vi "Setup JJ IV.vi"(4 "Channel Name (1)":u16(ring)=1 items=["1"=1, "2"=2, "3"=3, "4"=4], 5 "VISA resource name":refnum<visa-resource-name>="GPIB0::1::INSTR", 7 "End time S":dbl=0.000105, 8 "error in (no error)":errorcluster, 9 "Ramp time S":dbl=0.01, 10 "Delay time S":dbl=0.01, 11 "Sampling Frequency (Hz)":u64=10000000 format="%^.2e") -> (0 "error out":errorcluster)   [LabVIEW 2021]
uses:
  <instrlib>/Tektronix AWG 5000 7000 Series/Public/Configure/Channel/Assign Output Waveform (From Waveform List).vi
  <instrlib>/Tektronix AWG 5000 7000 Series/Public/Configure/Configure Output Timing (Sampling Frequency).vi
  <instrlib>/Tektronix AWG 5000 7000 Series/Tektronix AWG 5000 7000 Series.lvlib
panel:
  in  "Jump height over Vpp":dbl=0.05
  in  "Ramp time S 2":dbl=0.0005
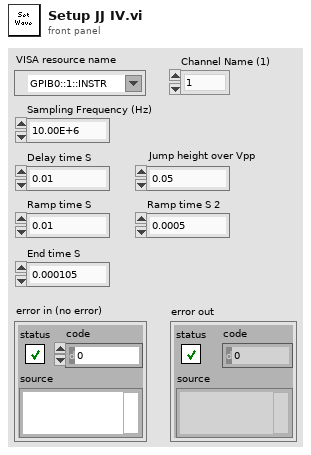
[diagram p1: front panel]
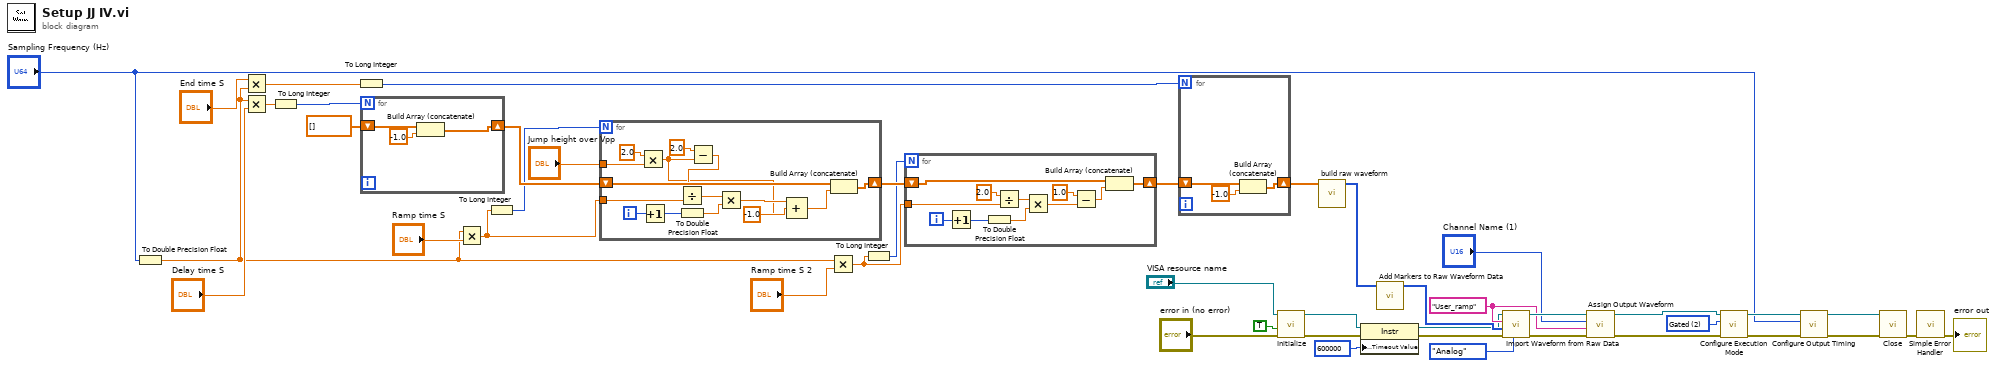
[diagram p0: block diagram]
diagram:
  w21 = u16 2 items=["Continuous", "Triggered", "Gated", "Sequence", "Triggered Continuous"] ("Execution Mode (0 : Continuous)")
  w23 = "User_ramp" ("Waveform Name")
  n1 = To Double Precision Float(number="Sampling Frequency (Hz)") -> (double precision float=w9:dbl)
  n2 = Multiply(x="End time S", y=w9) -> (x*y=w26:dbl)
  n3 = Multiply(x=w9, y="Delay time S") -> (x*y=w27:dbl)
  n4 = To Long Integer(number=w27) -> (32bit integer=w19:i32)
  n5 = To Long Integer(number=w26) -> (32bit integer=w2:i32)
  n6 = for {
    N: w19 -> [_]
    shift-right: [w46] -> w32
    shift-left: dbl[] [] -> [w47]
    n7 = Build Array (concatenate)(w47, -1.0) -> (w46:dbl[])
  }
  n8 = Multiply(x=w9, y="Ramp time S") -> (x*y=w5:dbl)
  n9 = To Long Integer(number=w5) -> (32bit integer=w18:i32)
  n10 = for {
    N: w18 -> [_]
    shift-right: [w55] -> w7
    shift-left: w32 -> [w57]
    tunnel: w5 -> [w54]
    tunnel: "Jump height over Vpp" -> [w51]
    i -> [w61]
    n11 = Multiply(x=2.0, y=w51) -> (x*y=w48:dbl)
    n12 = Increment(x=w61) -> (x+1=w60:i32)
    n13 = To Double Precision Float(number=w60) -> (double precision float=w53:dbl)
    n14 = Subtract(x=2.0, y=w48) -> (x-y=w49:dbl)
    n15 = Divide(x=w49, y=w54) -> (x/y=w62:dbl)
    n16 = Multiply(x=w62, y=w53) -> (x*y=w59:dbl)
    n17 = Compound Arithmetic op=ADD(w59, -1.0 ("y"), w48) -> (w56:dbl)
    n18 = Build Array (concatenate)(w57, w56) -> (w55:dbl[])
  }
  n19 = Multiply(x=w9, y="Ramp time S 2") -> (x*y=w4:dbl)
  n20 = To Long Integer(number=w4) -> (32bit integer=w3:i32)
  n21 = for {
    N: w3 -> [_]
    shift-right: [w72] -> w6
    shift-left: w7 -> [w73]
    tunnel: w4 -> [w71]
    i -> [w69]
    n22 = Increment(x=w69) -> (x+1=w68:i32)
    n23 = To Double Precision Float(number=w68) -> (double precision float=w66:dbl)
    n24 = Divide(x=2.0, y=w71) -> (x/y=w67:dbl)
    n25 = Multiply(x=w67, y=w66) -> (x*y=w64:dbl)
    n26 = Subtract(x=1.0, y=w64) -> (x-y=w63:dbl)
    n27 = Build Array (concatenate)(w73, w63) -> (w72:dbl[])
  }
  n28 = for {
    N: w2 -> [_]
    shift-right: [w75] -> w28
    shift-left: w6 -> [w76]
    n29 = Build Array (concatenate)(w76, -1.0) -> (w75:dbl[])
  }
  n30 = call <instrlib>:"Initialize.vi"("error in (no error)"="error in (no error)", "Reset (False)"=TRUE ("Reset? (F: No)"), "VISA resource name"="VISA resource name") -> ("error out"=w12:errorcluster, "VISA resource name out"=w14:refnum<visa-resource-name>)  [unwired: 7 in]
  n31 = call "build raw waveform.vi"("Y"=w28) -> ("Raw Waveform Data"=w17:u8[])  [unwired: 10 in]
  n32 = property class="Instr"(reference=w14, error in=w12, "General Settings:Timeout Value"=u32 600000) -> (reference out=w13:refnum<visa-resource-name>, error out=w11:errorcluster)
  n33 = call <instrlib>:"Add Markers to Raw Waveform Data.vi"("Raw Waveform Data"=w17) -> ("Raw Waveform Data with Markers"=w16:u8[])  [unwired: 10 in]
  n34 = call <instrlib>:"Import Waveform from Raw Data.vi"("Representation (1 : Analog)"=enum16{"Integer", "Analog"}."Analog", "error in (no error)"=w11, "Raw Data"=w16, "Waveform Name"=w23, "VISA resource name"=w13) -> ("error out"=w22:errorcluster, "VISA resource name out"=w24:refnum<visa-resource-name>)  [unwired: 5 in]
  n35 = call-poly <instrlib>:"Assign Output Waveform.vi"("error in (no error)"=w22, "Waveform"=w23, "Channel Name (1)"="Channel Name (1)", "VISA resource name"=w24) -> ("error out"=w42:errorcluster, "VISA resource name out"=w43:refnum<visa-resource-name>)  [unwired: 6 in]
  n36 = call <instrlib>:"Configure Execution Mode.vi"("error in (no error)"=w42, "Execution Mode (0 : Continuous)"=w21, "VISA resource name"=w43) -> ("error out"=w40:errorcluster, "VISA resource name out"=w41:refnum<visa-resource-name>)  [unwired: 7 in]
  n37 = call-poly <instrlib>:"Configure Output Timing.vi"("error in (no error)"=w40, "Sampling Frequency (Hz) (100MHz)"="Sampling Frequency (Hz)", "VISA resource name"=w41) -> ("error out"=w38:errorcluster, "VISA resource name out"=w39:refnum<visa-resource-name>)  [unwired: 7 in]
  n38 = call <instrlib>:"Close.vi"("error in (no error)"=w38, "VISA resource name"=w39) -> ("error out"=w37:errorcluster)  [unwired: 9 in]
  n39 = call <vilib>:"Simple Error Handler.vi"("error in (no error)"=w37) -> ("error out"=→"error out":errorcluster)  [unwired: 4 in, 4 out]
